vi "Define Test Suite (Default).vi"(4 "timeout":i32=2000, 6 "Verbose (F)":bool, 7 "Test Report (optional)":refnum<class "Test Report.lvclass">, 8 "error in (no error)":errorcluster, 10 "Interactive":bool, 11 "Label (VI Title)":string) -> (0 "error out":errorcluster, 2 "Properties.Suite":refnum<class "Properties.Suite.lvclass">, 3 "Test Suite":refnum<class "Test Suite.lvclass">)   [LabVIEW 2013, in "Caraya.lvlib" / "Test Suite.lvclass"]
doc: "Registers the calling VI as a test suite. If Interactive is True, the interactive user interface is opened when the test suite is executed. If the Report Path is set, a report file will be generated with the test results.\n\n--\nCopyright © 2015 JKI All rights reserved.\n\nAuthor: Tomi Maila <tomi.maila@jki.net>\n\nThis library is provided \"AS IS\" ,WITHOUT WARRANTIES OR\nCONDITIONS OF ANY KIND, either express or implied.\n\nJKI -- jki.net"
uses:
  Test Suite.lvclass
  Test Report/Test Report.lvclass
  Properties.Suite/Properties.Suite.lvclass
  Test Assert Factory/Test Assert Factory.lvclass
  Test Suite.lvclass/Test Suite.ctl
  Properties.Suite/Properties.Suite.lvclass/Properties.Suite.ctl
  Caraya.lvlib
  Assert Factory Manager/Assert Factory Manager.lvclass
  Basic Test Manager/Basic Test Manager.lvclass
  Properties/Properties.lvclass
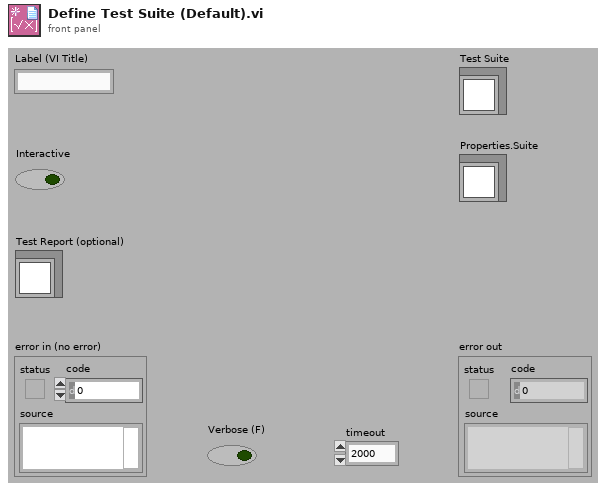
[diagram p1: front panel]
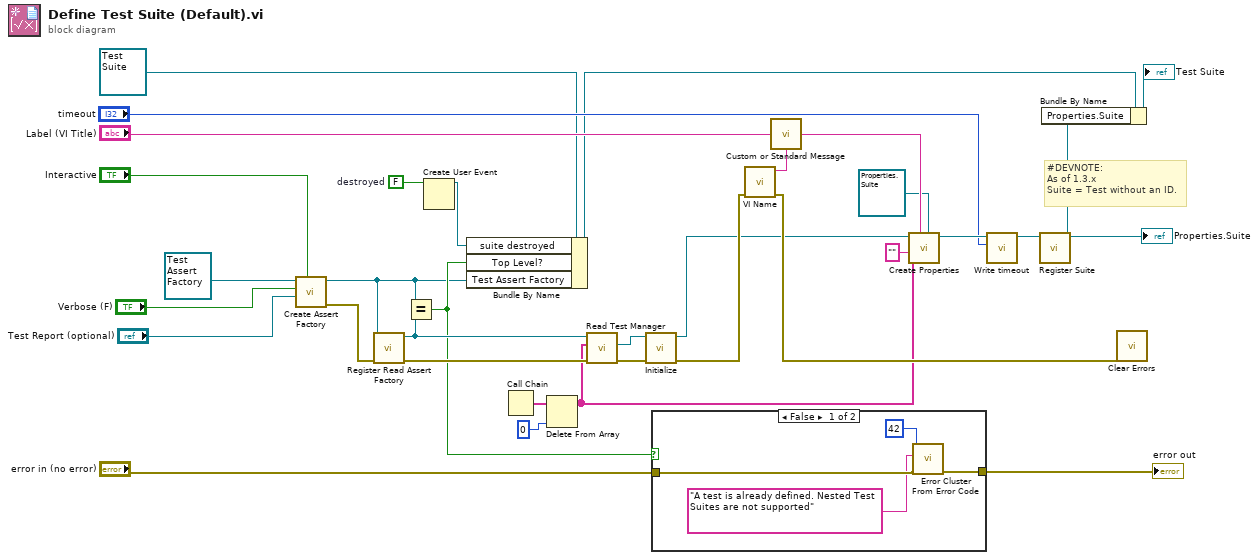
[diagram p0: block diagram]
diagram:
  w14 = FALSE  # destroyed
  # "#DEVNOTE:\nAs of 1.3.x\nSuite = Test without an ID."
  n1 = call "Create Assert Factory.vi"("Interactive"="Interactive", "Test Report"="Test Report (optional)", "Verbose (F)"="Verbose (F)", "Test Assert Factory in"=refnum<class "Test Assert Factory.lvclass"> refnum ("Caraya.lvlib:Test Assert Factory.lvclass")) -> ("error out"=w17:errorcluster, "Test Assert Factory out"=w18:refnum<class "Test Assert Factory.lvclass">)  [unwired: 6 in]
  n2 = call "Register Read Assert Factory.vi"("error in (no error)"=w17, "Test Assert Factory"=w18) -> ("error out"=w32:errorcluster, "Test Assert Factory"=w25:refnum<class "Test Assert Factory.lvclass">)  [unwired: 8 in]
  n3 = Equal?(x=w18, y=w25) -> (x = y?=w22:bool)
  n4 = Create User Event(user event datatype=w14) -> (user event=w13:refnum<user-event>)  [unwired: 1 in, 1 out]
  n5 = Bundle By Name(cluster=refnum<class "Test Suite.lvclass"> refnum ("Test Suite"), "suite destroyed"=w13, "Top Level?"=w22, "Test Assert Factory"=w18) -> (w2:refnum<class "Test Suite.lvclass">)
  n6 = Call Chain() -> (call chain=w26:string[])
  n7 = Delete From Array(array=w26, index=0) -> (array with subset deleted=w8:string[])  [unwired: 1 in, 1 out]
  n8 = call-dynamic "Read Test Manager.vi"("error in (no error)"=w32, "VI Call Chain"=w8, "Assert Factory in"=w25) -> ("error out"=w30:errorcluster, "Basic Test Manager"=w21:refnum<class "Basic Test Manager.lvclass">)  [unwired: 6 in, 1 out]
  n9 = call "Initialize.vi"("error in (no error)"=w30, "Test Manager in"=w21) -> ("error out"=w29:errorcluster, "Test Manager out"=w12:refnum<class "Basic Test Manager.lvclass">)  [unwired: 8 in]
  n10 = case shown="False" w22 {
    tunnel: [w37 w38] -> w24
    tunnel: "error in (no error)" -> [w36 w38]
    frame False {
      n11 = call <vilib>:"Error Cluster From Error Code.vi"("error in (no error)"=w36, "error message (\"\")"="A test is already defined. Nested Test Suites are not supported" ("error message (\"\")"), "error code (0)"=42) -> ("error out"=w37:errorcluster)  [unwired: 6 in]
    }
    frame True {
    }
  }
  "error out" <- w24
  n12 = call "VI Name.vi"("error in (no error)"=w29) -> ("error out"=w28:errorcluster, "VI Name"=w31:string)  [unwired: 9 in]
  n13 = call "Custom or Standard Message.vi"("Custom Message"="Label (VI Title)", "Standard Message"=w31) -> ("Message"=w11:string)
  n14 = call "Create Properties.vi"("Properties in"=refnum<class "Properties.Suite.lvclass"> refnum ("Caraya.lvlib:Properties.Suite.lvclass"), "label"=w11, "call-chain"=w8, "self-id"="", "Test Manager"=w12) -> ("Properties out"=w7:refnum<class "Properties.Suite.lvclass">)  [unwired: 6 in]
  n15 = call "Write timeout.vi"("timeout"="timeout", "Properties.Suite in"=w7) -> ("Properties.Suite out"=w6:refnum<class "Properties.Suite.lvclass">)  [unwired: 9 in]
  n16 = call "Register Suite.vi"("Properties.Suite in"=w6) -> ("Properties.Suite out"=w3:refnum<class "Properties.Suite.lvclass">)  [unwired: 10 in]
  "Properties.Suite" <- w3
  n17 = Bundle By Name(cluster=w2, "Properties.Suite"=w3) -> (→"Test Suite":refnum<class "Test Suite.lvclass">)
  n18 = call <vilib>:"Clear Errors.vi"("error in (no error)"=w28) -> ()  [unwired: 6 in, 1 out]
